vi "Update_STS_Param_Data_SubVI.vi"(11 "STSparameters":T1) -> ()   [LabVIEW 2014]
uses:
  <userlib>/Nanonis Prog Interface V5/Nanonis Prog Interface.lvlib
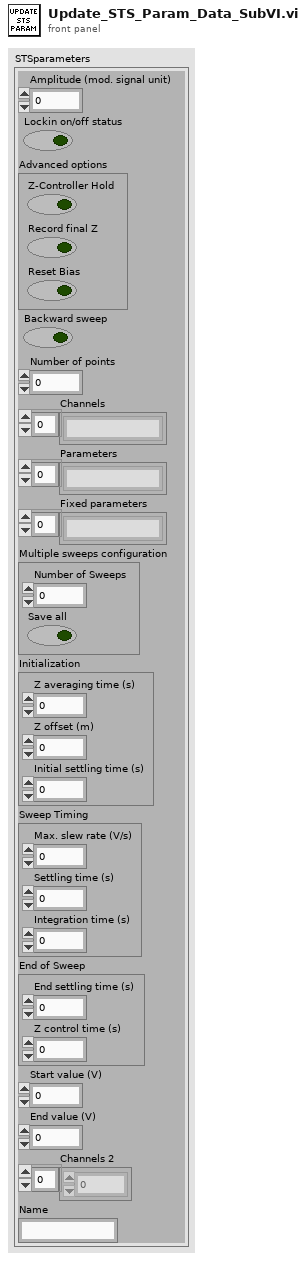
[diagram p1: front panel]
types:
  T1 = cluster{"Amplitude (mod. signal unit)":sgl, "Lockin on/off status":bool, "Advanced options":cluster{"Z-Controller Hold":bool, "Record final Z":bool, "Reset Bias":bool}, "Backward sweep":bool, "Number of points":i32, "Channels":string[], "Parameters":string[], "Fixed parameters":string[], "Multiple sweeps configuration":cluster{"Number of Sweeps":i32, "Save all":bool}, "Initialization":cluster{"Z averaging time (s)":sgl, "Z offset (m)":sgl, "Initial settling time (s)":sgl}, "Sweep Timing":cluster{"Max. slew rate (V/s)":sgl, "Settling time (s)":sgl, "Integration time (s)":sgl}, "End of Sweep":cluster{"End settling time (s)":sgl, "Z control time (s)":sgl}, "Start value (V)":sgl, "End value (V)":sgl, "Channels 2":i32[], "Name":string}
  T2 = cluster{"Save all":enum16{"no change", "on", "off"}, "Number of Sweeps (0=no change)":i32}
  T3 = cluster{"Z-Controller Hold":bool, "Record final Z":bool, "Reset Bias":bool}
  T4 = cluster{"Z averaging time (s)":sgl, "Z offset (m)":sgl, "Initial settling time (s)":sgl}
  T5 = cluster{"Max. slew rate (V/s)":sgl, "Settling time (s)":sgl, "Integration time (s)":sgl}
  T6 = cluster{"End settling time (s)":sgl, "Z control time (s)":sgl}
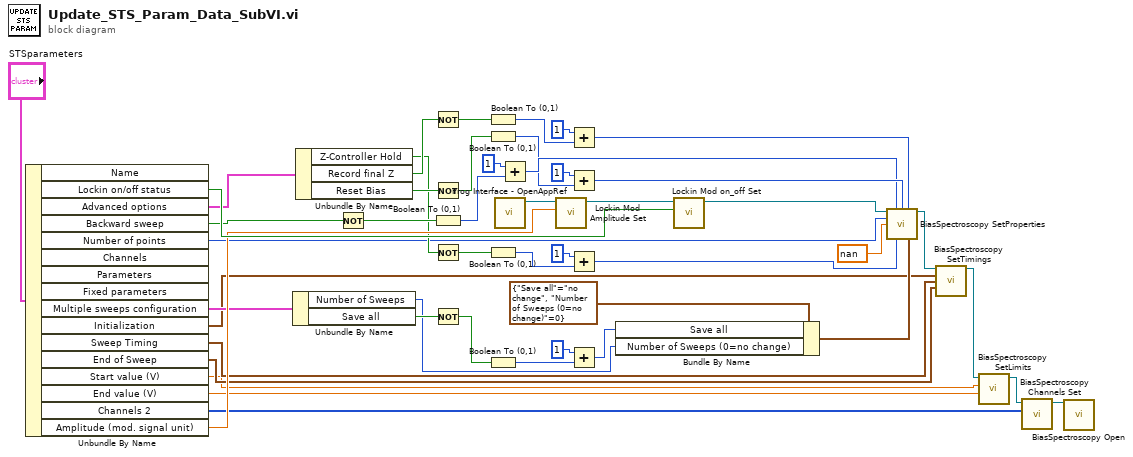
[diagram p0: block diagram]
diagram:
  n1 = Unbundle By Name("STSparameters") -> ("Lockin on/off status"=w47:bool, "Advanced options"=w13:T3, "Backward sweep"=w14:bool, "Number of points"=w11:i32, "Multiple sweeps configuration"=w12:cluster{"Number of Sweeps":i32, "Save all":bool}, "Initialization"=w10:T4, "Sweep Timing"=w9:T5, "End of Sweep"=w8:T6, "Start value (V)"=w6:sgl, "End value (V)"=w7:sgl, "Channels 2"=w5:i32[], "Amplitude (mod. signal unit)"=w37:sgl)  [unwired: 4 out]
  n2 = Unbundle By Name(w12) -> ("Number of Sweeps"=w26:i32, "Save all"=w30:bool)
  n3 = Unbundle By Name(w13) -> ("Z-Controller Hold"=w21:bool, "Record final Z"=w22:bool, "Reset Bias"=w25:bool)
  n4 = Not(x=w14) -> (.not. x?=w34:bool)
  n5 = Not(x=w22) -> (.not. x?=w32:bool)
  n6 = Not(x=w25) -> (.not. x?=w33:bool)
  n7 = Boolean To (0,1)(Boolean=w34) -> (0, 1=w15:i16)
  n8 = Not(x=w21) -> (.not. x?=w35:bool)
  n9 = Not(x=w30) -> (.not. x?=w36:bool)
  n10 = Boolean To (0,1)(Boolean=w32) -> (0, 1=w17:i16)
  n11 = Boolean To (0,1)(Boolean=w33) -> (0, 1=w23:i16)
  n12 = Boolean To (0,1)(Boolean=w35) -> (0, 1=w19:i16)
  n13 = Boolean To (0,1)(Boolean=w36) -> (0, 1=w27:i16)
  n14 = call <userlib>:"Prog Interface - OpenAppRef.vi"() -> ("Application reference"=w48:refnum<vi>)  [unwired: 6 in, 1 out]
  n15 = Add(x=i16 1, y=w15) -> (x+y=w38:i16)
  n16 = call <userlib>:"Lockin Mod Amplitude Set.vi"("Amplitude (mod. signal unit)"=w37, "Application ref in"=w48) -> ("Application ref out"=w2:refnum<vi>)  [unwired: 8 in, 1 out]
  n17 = Add(x=i16 1, y=w17) -> (x+y=w45:i16)
  n18 = Add(x=i16 1, y=w23) -> (x+y=w41:i16)
  n19 = Add(x=i16 1, y=w19) -> (x+y=w46:i16)
  n20 = Add(x=i16 1, y=w27) -> (x+y=w29:i16)
  n21 = Bundle By Name(cluster=T2 {"Save all"=enum."no change", "Number of Sweeps (0=no change)"=0} ("Multiple sweeps config"), "Save all"=w29, "Number of Sweeps (0=no change)"=w26) -> (w43:T2)
  n22 = call <userlib>:"Lockin Mod on_off Set.vi"("Lockin ON/OFF"=w47, "Application ref in"=w2) -> ("Application ref out"=w39:refnum<vi>)  [unwired: 8 in, 1 out]
  n23 = call <userlib>:"BiasSpectroscopy SetProperties.vi"("Application ref in"=w39, "Backward sweep (no change)"=w38, "Reset Bias (no change)"=w41, "Record final Z position"=w45, "Number of points (0=no change)"=w11, "Z offset (m) (NaN=no change)"=sgl nan, "Z-Controller hold (no change)"=w46, "Multiple sweeps config"=w43) -> ("Application ref out"=w40:refnum<vi>)  [unwired: 6 in, 1 out]
  n24 = call <userlib>:"BiasSpectroscopy SetTimings.vi"("Application ref in"=w40, "Initialization (NaN)"=w10, "Sweep Timing (NaN)"=w9, "End of Sweep (NaN)"=w8) -> ("Application ref out"=w3:refnum<vi>)  [unwired: 10 in, 1 out]
  n25 = call <userlib>:"BiasSpectroscopy SetLimits.vi"("End value (V)"=w7, "Start value (V)"=w6, "Application ref in"=w3) -> ("Application ref out"=w4:refnum<vi>)  [unwired: 5 in, 1 out]
  n26 = call <userlib>:"BiasSpectroscopy Channels Set.vi"("Channels"=w5, "Application ref in"=w4) -> ("Application ref out"=w31:refnum<vi>)  [unwired: 8 in, 1 out]
  n27 = call <userlib>:"BiasSpectroscopy Open.vi"("Application ref in"=w31) -> ()  [unwired: 13 in, 2 out]
